vi "Update.vi"(8 "error in (no error)":errorcluster, 10 "Value":dbl, 11 "dY_dX_Calculator in":refnum<class "delayValue.lvclass">) -> (0 "error out":errorcluster, 3 "dY_dX_Calculator out":refnum<class "delayValue.lvclass">)   [LabVIEW 2019, in "delayValue.lvclass"]
uses:
  delayValue.lvclass
  delayValue.lvclass/delayValue.ctl
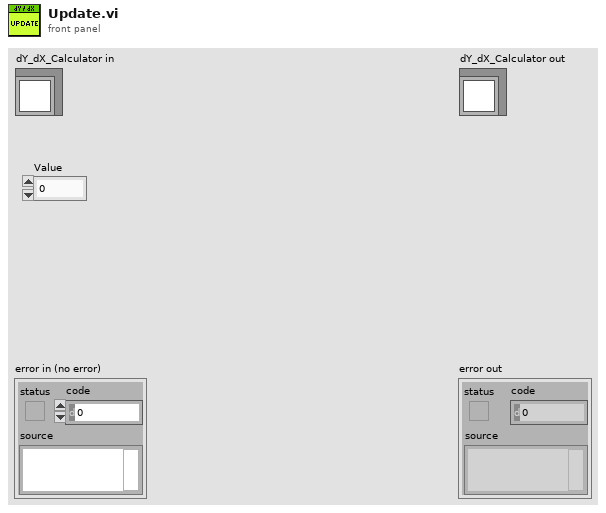
[diagram p1: front panel]
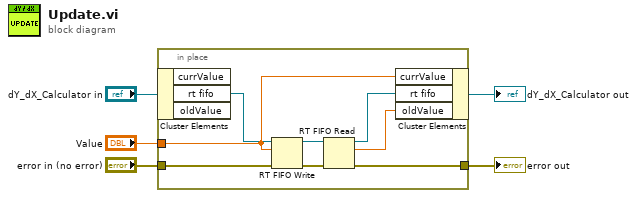
[diagram p0: block diagram]
diagram:
  n1 = in-place {
    in-place-border: "Value" -> [w6]
    in-place-border: "error in (no error)" -> [w8]
    in-place-border: [w10] -> w1
    n2 = in-place-cluster #1("dY_dX_Calculator in") -> ("rt fifo"=w12:refnum<k33>)  [unwired: 2 out]
    n3 = RT FIFO Write(0:w12, 1:w6, 3:w8) -> (8:w9:refnum<k33>, 11:w13:errorcluster)  [unwired: 2 in, 2 out]
    n4 = RT FIFO Read(0:w9, 3:w13) -> (8:w11:refnum<k33>, 9:w7:dbl, 11:w10:errorcluster)  [unwired: 2 in, 2 out]
    n5 = in-place-cluster #1("currValue"=w6, "rt fifo"=w11, "oldValue"=w7) -> (→"dY_dX_Calculator out":refnum<class "delayValue.lvclass">)
  }
  "error out" <- w1
